vi "NicmosGetFilter.vi"(9 "error in (no error)":errorcluster caption="error out (no error)") -> (0 "FILTER out":T1, 6 "error out":errorcluster)   [LabVIEW 2009]
uses:
  Controls/NICMOS.FILTER.ctl
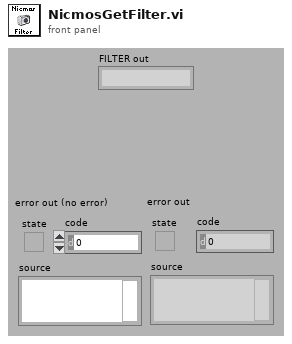
[diagram p1: front panel]
types:
  T1 = typedef "NICMOS.FILTER.ctl" = string
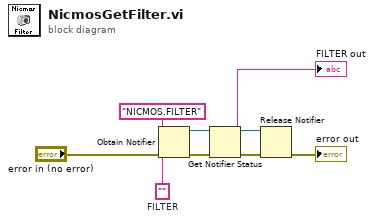
[diagram p0: block diagram]
diagram:
  w8 = T1 ""  # FILTER
  n1 = Obtain Notifier(name (unnamed)="NICMOS.FILTER" ("nom (aucun)"), notification data type=w8, error in (no error)="error in (no error)") -> (notifier out=w1:refnum<notifier>, error out=w2:errorcluster)  [unwired: 1 in, 1 out]
  n2 = Get Notifier Status(notifier=w1, error in (no error)=w2) -> (notifier out=w4:refnum<notifier>, current notification=→"FILTER out":T1, error out=w6:errorcluster)  [unwired: 2 out]
  n3 = Release Notifier(notifier=w4, error in (no error)=w6) -> (error out=→"error out":errorcluster)  [unwired: 1 in, 2 out]
